vi "CODCr启动 (子VI).vi"(11 "启动测量模式":T2) -> (0 "error out":T1={"status"=FALSE, "代码"=4, "source"=""} caption="错误输出" {"代码" items=["执行成功"=1, "执行失败，但不知道原因"=2, "命令请求条件错误"=3, "通讯超时"=4, "系统繁忙不能执行"=5, "系统故障"=6, "没有数据"=100]})   [LabVIEW 2016]
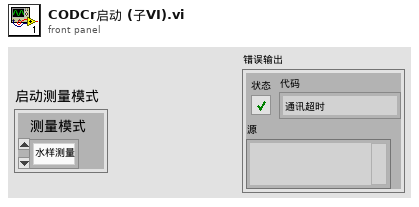
[diagram p1: front panel]
types:
  T1 = cluster{"status":bool, "代码":u16, "source":string}
  T2 = cluster{"测量模式":enum16{"水样测量", "标样核查", "零点核查", "跨度核查", "空白测试", "加标回收", "平行样", "校零", "校标"}}
  T3 = cluster{"命令":string, "测量模式":enum16{"水样测量", "标样核查", "零点核查", "跨度核查", "空白测试", "加标回收", "平行样", "校零", "校标"}, "CODMn量程切换":enum32{"H", "L", "AUTO"}}
  T4 = enum16{"水样测量", "标样核查", "零点核查", "跨度核查", "空白测试", "加标回收", "平行样", "校零", "校标"}
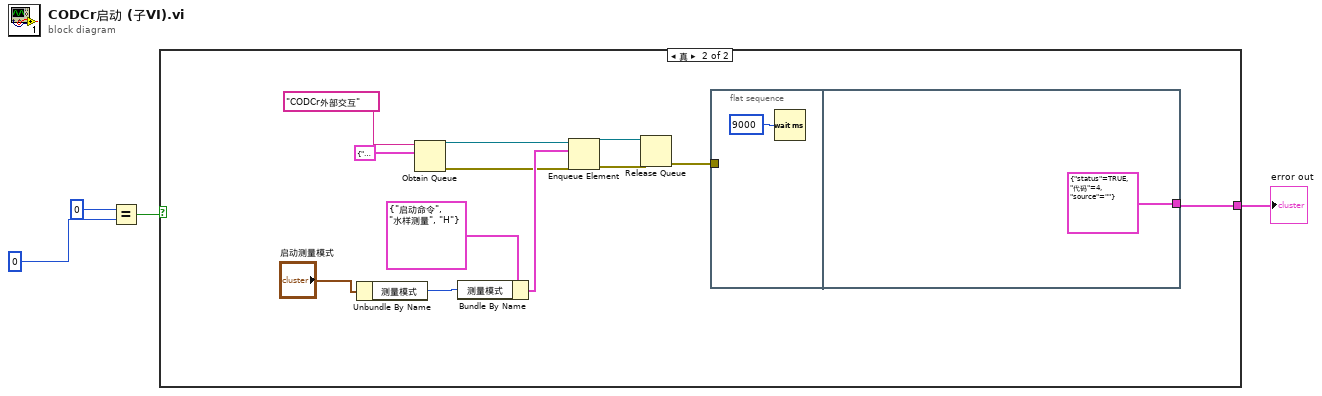
[diagram p0: block diagram]
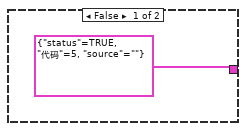
[diagram p2: hidden frame]
diagram:
  n1 = Equal?(x=u16 0, y=u16 0) -> (x = y?=w4:bool)
  n2 = case shown="真" w4 {
    tunnel: [T1 {"status"=TRUE, "代码"=5, "source"=""} ("error out") w6] -> w2
    frame False {
    }
    frame True {
      n3 = Unbundle By Name("启动测量模式") -> ("测量模式"=w8:T4)
      n4 = Obtain Queue(name (unnamed)="CODCr外部交互" ("名称（未命名）"), element data type=T3 {"命令"="启动命令", "测量模式"=enum."水样测量", "CODMn量程切换"=enum."AUTO"} ("元素")) -> (queue out=w11:refnum<queue>, error out=w10:errorcluster)  [unwired: 3 in, 1 out]
      n5 = Bundle By Name(cluster=T3 {"命令"="启动命令", "测量模式"=enum."水样测量", "CODMn量程切换"=enum."H"} ("元素"), "测量模式"=w8) -> (w12:T3)
      n6 = Enqueue Element(queue=w11, element=w12, error in (no error)=w10) -> (queue out=w15:refnum<queue>, error out=w14:errorcluster)  [unwired: 1 in, 1 out]
      n7 = Release Queue(queue=w15, error in (no error)=w14) -> (error out=w7:errorcluster)  [unwired: 1 in, 2 out]
      n8 = flat-sequence {
        tunnel: w7 -> [_]
        tunnel: [T1 {"status"=TRUE, "代码"=4, "source"=""} ("error out")] -> w6
        frame #0 {
          n9 = Wait (ms)(milliseconds to wait=u32 9000 ("等待时间（毫秒）")) -> ()  [unwired: 1 out]
        }
        frame #1 {
        }
      }
    }
  }
  "error out" <- w2
